vi "Omron_DM_Read.vi"(6 "No of Words":u16 max=9999 format="%04.0f", 7 "Beginning Words":u16 max=9999 format="%04.0f", 8 "error in":errorcluster, 9 "Command":string="RR", 10 "Unit No.":u8 max=31 format="%02.0f", 11 "COM in":refnum<visa-resource-name>) -> (0 "error out":errorcluster, 2 "Read Data":u32[](array[numeric]), 3 "COM out":refnum<visa-resource-name>)   [LabVIEW 2015]
panel:
  out "连接的字符串":string
  out "Response":string
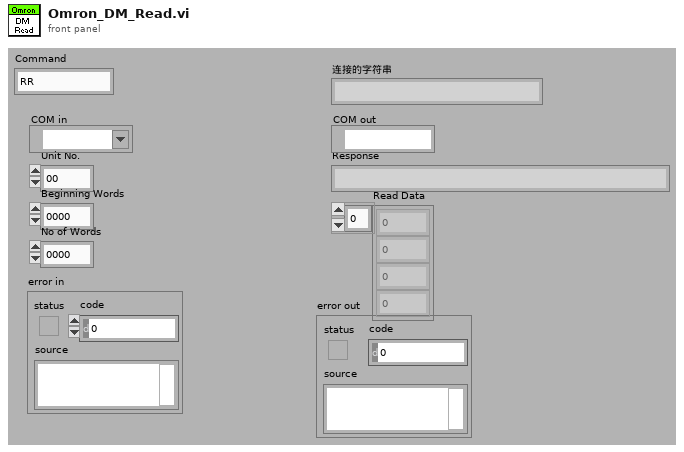
[diagram p1: front panel]
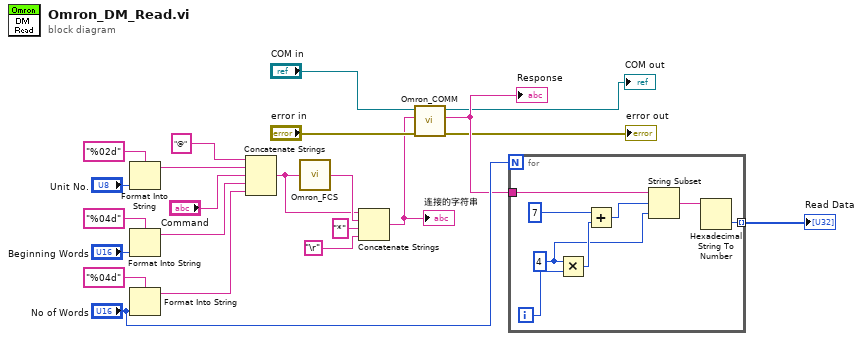
[diagram p0: block diagram]
diagram:
  n1 = Format Into String(format string="%02d", "Unit No.") -> (resulting string=w19:string)  [unwired: 2 in, 1 out]
  n2 = Format Into String(format string="%04d", "Beginning Words") -> (resulting string=w14:string)  [unwired: 2 in, 1 out]
  n3 = Format Into String(format string="%04d", "No of Words") -> (resulting string=w13:string)  [unwired: 2 in, 1 out]
  n4 = Concatenate Strings("@" ("Command"), w19, "Command", w14, w13) -> (w1:string)
  n5 = call "Omron_FCS.vi"("Command"=w1) -> ("FCS"=w12:string)
  n6 = Concatenate Strings(w1, w12, "*" ("string"), "\r") -> (w5:string)
  "连接的字符串" <- w5
  n7 = call "Omron_COMM.vi"("error in"="error in", "Write data"=w5, "COM in"="COM in") -> ("error out"=→"error out":errorcluster, "Receive data"=w4:string, "COM out"=→"COM out":refnum<visa-resource-name>)  [unwired: 6 in]
  "Response" <- w4
  n8 = for {
    N: "No of Words" -> [_]
    tunnel: w4 -> [w30]
    tunnel: [w23] -> w8 mode=indexing
    i -> [w29]
    w25 = 4 ("x")
    n9 = Multiply(x=w25, y=w29) -> (x*y=w28:i32)
    n10 = Add(x=7 ("offset (0)"), y=w28) -> (x+y=w26:i32)
    n11 = String Subset(string=w30, offset (0)=w26, length (rest)=w25) -> (substring=w24:string)
    n12 = Hexadecimal String To Number(string=w24) -> (number=w23:u32)  [unwired: 2 in, 1 out]
  }
  "Read Data" <- w8
